vi "getContext.vi"(8 "error in (no error)":errorcluster, 11 "IComponent in":refnum<class "IComponent.lvclass">) -> (0 "error out":errorcluster, 2 "Context out":refnum<class "IContext.lvclass">, 3 "IComponent out":refnum<class "IComponent.lvclass">)   [LabVIEW 2022 SP3, in "openDAQ.lvlib" / "IBaseObject.lvlib" / "IPropertyObject.lvlib" / "IComponent.lvlib" / "IComponent.lvclass"]
uses:
  <instrlib>/openDAQ/Public/Classes/IComponent/IComponent.lvclass
  <instrlib>/openDAQ/Public/Classes/IComponent/IComponent.lvclass/IComponent.ctl
  <instrlib>/openDAQ/Public/Classes/IContext/IContext.lvclass
  <instrlib>/openDAQ/Binaries/Windows/x86/copendaq32.dll
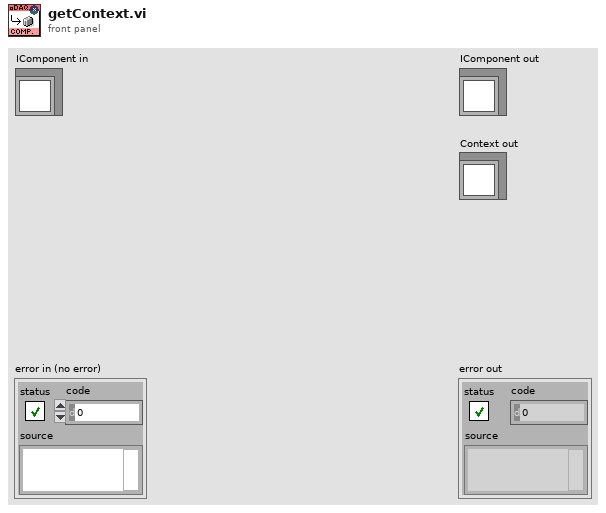
[diagram p1: front panel]
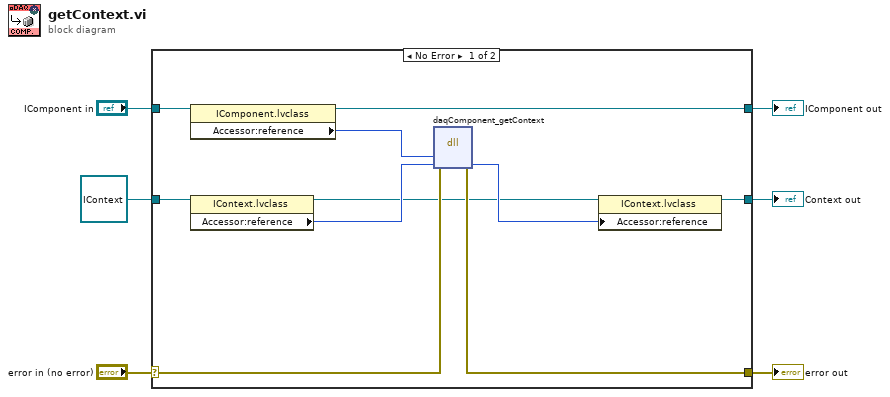
[diagram p0: block diagram]
diagram:
  n1 = case shown="No Error" "error in (no error)" {
    selector: "error in (no error)" -> [w11 w19]
    tunnel: [w14 w19] -> w5
    tunnel: [w12 w18] -> w3
    tunnel: "IComponent in" -> [w13 w18]
    tunnel: [w8 w17] -> w1
    tunnel: refnum<class "IContext.lvclass"> refnum ("openDAQ.lvlib:IBaseObject.lvlib:IContext.lvlib:IContext.lvclass") -> [w7 w17]
    frame No Error {
      n2 = property class="IComponent.lvclass"(reference=w13) -> (reference out=w12:refnum<class "IComponent.lvclass">, "Accessor:reference"=w9:i64)  [unwired: 1 in, 1 out]
      n3 = property class="IContext.lvclass"(reference=w7) -> (reference out=w10:refnum<class "IContext.lvclass">, "Accessor:reference"=w15:i64)  [unwired: 1 in, 1 out]
      n4 = dll-call lib="C:/Program Files (x86)/National Instruments/LabVIEW 2022/instr.lib/openDAQ/Binaries/Windows/x86/copendaq*.*" fn="daqComponent_getContext"(error in=w11, "component"=w9, "context"=w15) -> (error out=w14:errorcluster, "context"=w16:i64)  [unwired: 4 in, 1 out]
      n5 = property class="IContext.lvclass"(reference=w10, "Accessor:reference"=w16) -> (reference out=w8:refnum<class "IContext.lvclass">)  [unwired: 1 in, 1 out]
    }
    frame Error {
    }
  }
  "error out" <- w5
  "IComponent out" <- w3
  "Context out" <- w1
